vi "ex_3.vi"() -> ()   [LabVIEW 2020]
panel:
  out "y'":i32[](array[numeric])
  out "XY Graph":cluster{i32[], i32[]}(graph)
  out "y":i32[](array[numeric])
  out "x":i32[](array[numeric])
  in  "Longest side of spiral":i32
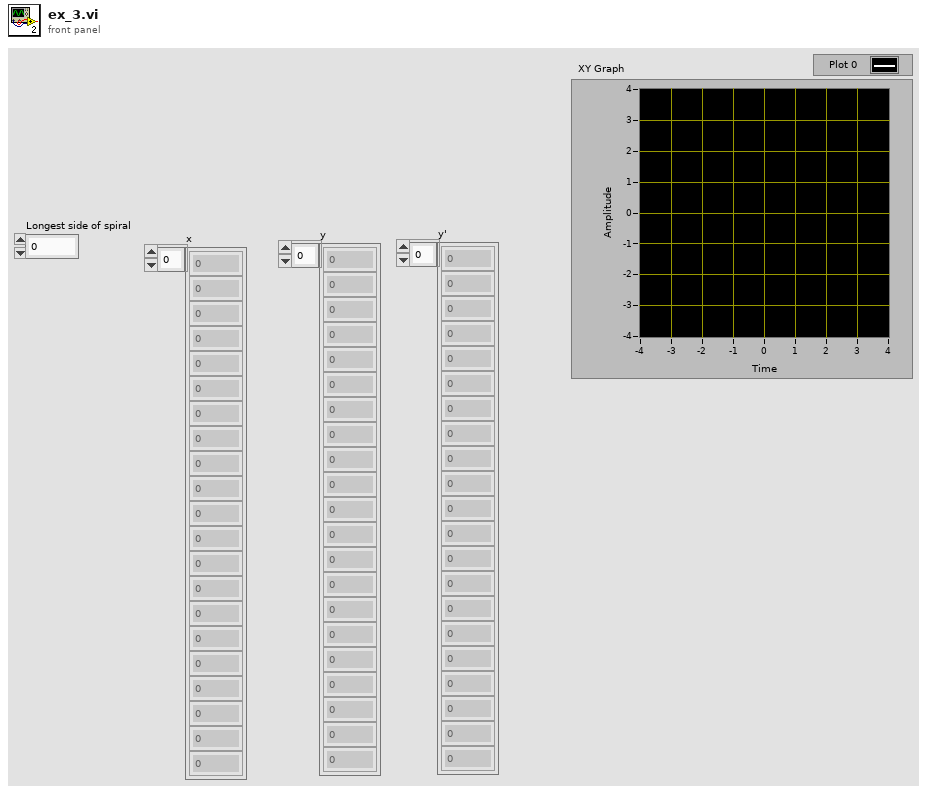
[diagram p1: front panel]
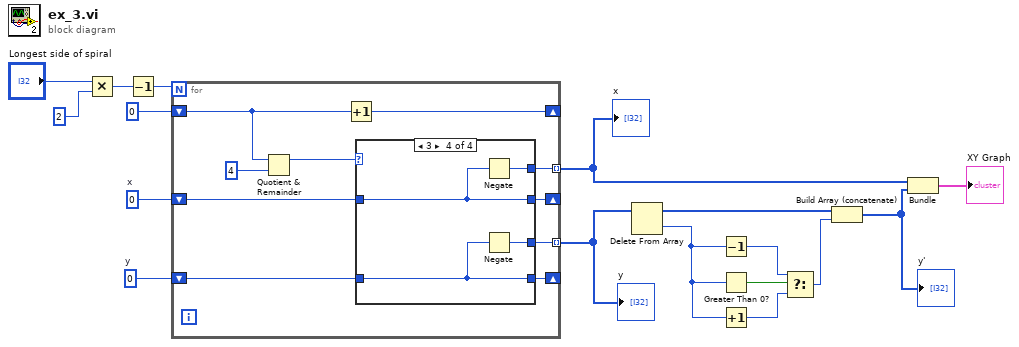
[diagram p0: block diagram]
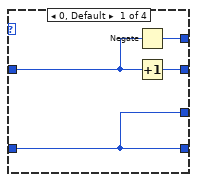
[diagram p2: hidden frame]
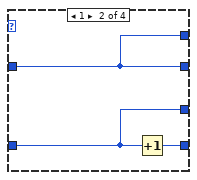
[diagram p3: hidden frame]
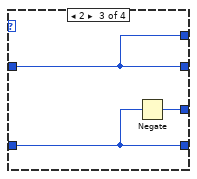
[diagram p4: hidden frame]
diagram:
  w12 = 0  # y
  w13 = 0  # x
  n1 = Multiply(x="Longest side of spiral", y=2) -> (x*y=w15:i32)
  n2 = Decrement(x=w15) -> (x-1=w1:i32)
  n3 = for {
    N: w1 -> [_]
    shift-right: [w27] -> _
    shift-left: 0 -> [w19]
    shift-right: [w24] -> _
    shift-left: w13 -> [w26]
    shift-right: [w23] -> _
    shift-left: w12 -> [w25]
    tunnel: [w22] -> w11 mode=indexing
    tunnel: [w21] -> w3 mode=indexing
    n4 = Quotient & Remainder(x=w19, y=4) -> (x-y*floor(x/y)=w18:i32)  [unwired: 1 out]
    n5 = Increment(x=w19) -> (x+1=w27:i32)
    n6 = case shown="3" w18 {
      tunnel: w26 -> [w30 w34 w36 w40]
      tunnel: w25 -> [w31 w32 w37 w41]
      tunnel: [w29 w34 w36 w40] -> w24
      tunnel: [w31 w33 w37 w41] -> w23
      tunnel: [w28 w34 w36 w39] -> w22
      tunnel: [w31 w32 w35 w38] -> w21
      frame 0, Default {
        n7 = Negate(x=w30) -> (-x=w28:i32)
        n8 = Increment(x=w30) -> (x+1=w29:i32)
      }
      frame 1 {
        n9 = Increment(x=w32) -> (x+1=w33:i32)
      }
      frame 2 {
        n10 = Negate(x=w37) -> (-x=w35:i32)
      }
      frame 3 {
        n11 = Negate(x=w40) -> (-x=w39:i32)
        n12 = Negate(x=w41) -> (-x=w38:i32)
      }
    }
  }
  "x" <- w11
  "y" <- w3
  n13 = Delete From Array(array=w3) -> (deleted portion=w7:i32, array with subset deleted=w5:i32[])  [unwired: 2 in]
  n14 = Decrement(x=w7) -> (x-1=w8:i32)
  n15 = Greater Than 0?(x=w7) -> (x > 0?=w9:bool)
  n16 = Increment(x=w7) -> (x+1=w6:i32)
  n17 = Select(t=w8, s=w9, f=w6) -> (s? t:f=w2:i32)
  n18 = Build Array (concatenate)(w5, w2) -> (w4:i32[])
  "y'" <- w4
  n19 = Bundle(w11, w4) -> (→"XY Graph":cluster{i32[], i32[]})  [unwired: 1 in]
